vi "Did Interval Elapse.vi"(3 "Future time coordinate (ms)":u32) -> (0 "ms Until Next":dbl, 1 "Interval Elapsed?":bool)   [LabVIEW 2021, in "Interval Timer.lvlib"]
doc: "Given the 'Future time coordinate (ms)', return TRUE for 'Interval Elapsed?' if the current time is later. Otherwise, return FALSE and the remaining time to pass in 'ms Until Next'."
uses:
  Interval Timer.lvlib
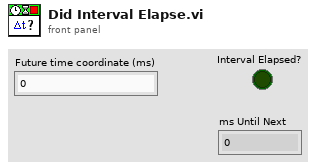
[diagram p1: front panel]
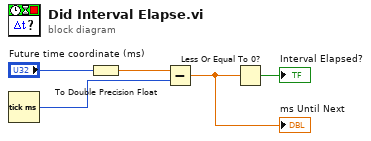
[diagram p0: block diagram]
diagram:
  n1 = Tick Count (ms)() -> (millisecond timer value=w4:u32)
  n2 = To Double Precision Float(number="Future time coordinate (ms)") -> (double precision float=w1:dbl)
  n3 = Subtract(x=w1, y=w4) -> (x-y=w3:dbl)
  "ms Until Next" <- w3
  n4 = Less Or Equal To 0?(x=w3) -> (x <= 0?=→"Interval Elapsed?":bool)
